vi "LinkTest.vi"(11 "number of nodes":i32) -> (3 "summary":T1[](array[typedef]))   [LabVIEW 2013, in "NISE_CEF_Tests.lvlib"]
uses:
  Trunk/CEF_TreeControl/Node/Summary.ctl
  Trunk/ProjectTemplates/Source/Configuration Editor Framework/Classes/cRIO/cRIO.lvclass
  Trunk/ProjectTemplates/Source/Configuration Editor Framework/Classes/cRIO/cRIO.lvclass/cRIO.ctl
  Trunk/ProjectTemplates/Source/Configuration Editor Framework/Classes/cRIO/Write System Name.vi
  NISE_CEF_Tests.lvlib
  Trunk/CEF_TreeControl/NISE_CEF_TreeControl.lvlib
  Trunk/CEF_TreeControl/Node/NISE_CEF_Node.lvclass
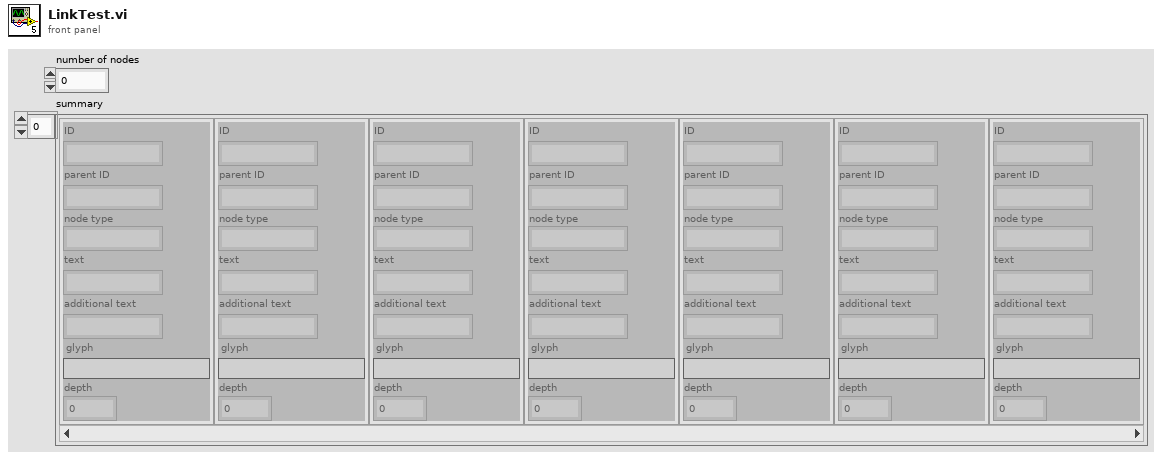
[diagram p1: front panel]
types:
  T1 = typedef "NISE_CEF_Node.lvclass/Summary.ctl" = cluster{"ID":string, "parent ID":string, "node type":string, "text":string, "additional text":string, "glyph":string, "depth":i32}
  T2 = typedef "NISE_CEF_Node.lvclass/NodeRef.ctl" = refnum<data-value>
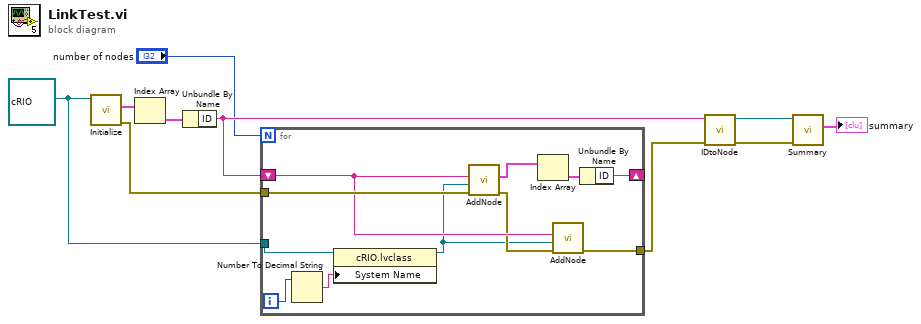
[diagram p0: block diagram]
diagram:
  w1 = refnum<class "cRIO.lvclass"> refnum ("cRIO.lvclass")
  n1 = call-dynamic "Initialize.vi"("cRIO in"=w1) -> ("error out"=w7:errorcluster, "summary"=w10:T1[])  [unwired: 8 in, 1 out]
  n2 = Index Array(array=w10) -> (element=w9:T1)  [unwired: 1 in]
  n3 = Unbundle By Name(w9) -> ("ID"=w8:string)
  n4 = for {
    N: "number of nodes" -> [_]
    tunnel: w1 -> [w14]
    shift-right: [w19] -> _
    shift-left: w8 -> [w17]
    tunnel: w7 -> [w18]
    tunnel: [w15] -> w3
    i -> [w13]
    n5 = Number To Decimal String(number=w13) -> (decimal integer string=w12:string)  [unwired: 1 in]
    n6 = property class="cRIO.lvclass"(reference=w14, "System Name"=w12) -> (reference out=w11:refnum<class "cRIO.lvclass">)  [unwired: 1 in, 1 out]
    n7 = call "AddNode.vi"("error in"=w18, "node in"=w11, "parent node ID"=w17) -> ("error out"=w16:errorcluster, "summary"=w20:T1[])  [unwired: 7 in]
    n8 = Index Array(array=w20) -> (element=w21:T1)  [unwired: 1 in]
    n9 = call "AddNode.vi"("error in"=w16, "node in"=w11, "parent node ID"=w17) -> ("error out"=w15:errorcluster)  [unwired: 7 in, 1 out]
    n10 = Unbundle By Name(w21) -> ("ID"=w19:string)
  }
  n11 = call "IDtoNode.vi"("error in"=w3, "ID"=w8) -> ("error out"=w2:errorcluster, "node ref"=w4:T2)  [unwired: 7 in, 1 out]
  n12 = call "Summary.vi"("error in"=w2, "node self ref"=w4) -> ("summary"=→"summary":T1[])  [unwired: 8 in, 1 out]
